vi "Extract Zip Archive.vi"(8 "error in (no error)":errorcluster, 11 "File":path=path "") -> (0 "error out":errorcluster, 3 "Unzipped files":path[](array[path]))   [LabVIEW 2020, in "binary_installation_tools.lvlib"]
uses:
  binary_installation_tools.lvlib
  <vilib>/zip/NI_Unzip.lvlib
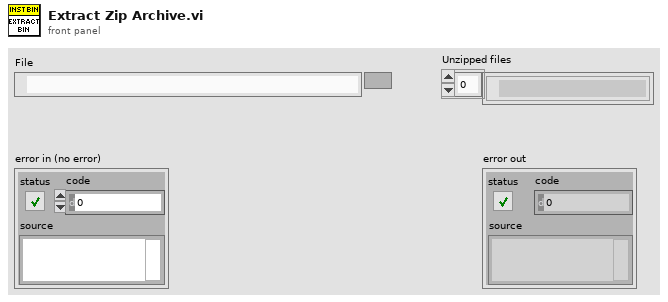
[diagram p1: front panel]
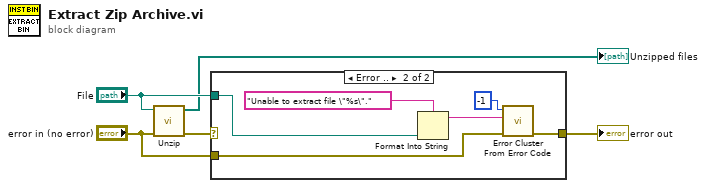
[diagram p0: block diagram]
diagram:
  n1 = call <vilib>:"Unzip.vi"("error in (no error)"="error in (no error)", "Zip file"="File") -> ("error out"=w3:errorcluster, "Unzipped files"=→"Unzipped files":path[])  [unwired: 7 in, 1 out]
  n2 = case shown="Error .." w3 {
    selector: w3 -> [w6 _]
    tunnel: [w6 w12] -> w5
    tunnel: "File" -> [_ w11]
    tunnel: "error in (no error)" -> [_ w7]
    frame No Error {
    }
    frame Error {
      n3 = Format Into String(format string="Unable to extract file \"%s\".", w11) -> (resulting string=w9:string)  [unwired: 2 in, 1 out]
      n4 = call <vilib>:"Error Cluster From Error Code.vi"("error in (no error)"=w7, "error message (\"\")"=w9, "error code (0)"=-1) -> ("error out"=w12:errorcluster)  [unwired: 6 in]
    }
  }
  "error out" <- w5
